vi "LiftSystem.vi"(11 "Lift System Actions":T1) -> ()   [LabVIEW 2019]
uses:
  Controls/Lift System Actions.ctl
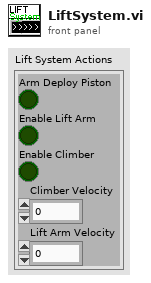
[diagram p1: front panel]
types:
  T1 = typedef "Lift System Actions.ctl" = cluster{"Arm Deploy Piston":bool, "Enable Lift Arm":bool, "Enable Climber":bool, "Climber Velocity":dbl, "Lift Arm Velocity":dbl}
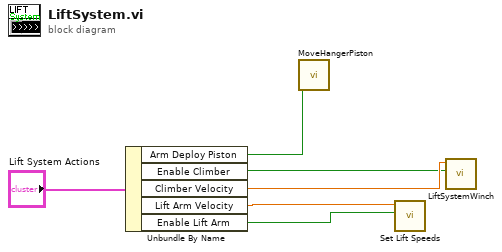
[diagram p0: block diagram]
diagram:
  n1 = Unbundle By Name("Lift System Actions") -> ("Arm Deploy Piston"=w1:bool, "Enable Climber"=w4:bool, "Climber Velocity"=w5:dbl, "Lift Arm Velocity"=w3:dbl, "Enable Lift Arm"=w2:bool)
  n2 = call "MoveHangerPiston.vi"("Arm Deploy Piston"=w1) -> ()  [unwired: 11 in]
  n3 = call "Set Lift Speeds.vi"("Enable Lift Arm"=w2, "Lift Speed"=w3) -> ()  [unwired: 10 in]
  n4 = call "LiftSystemWinch.vi"("Enable"=w4, "climber velocity"=w5) -> ()  [unwired: 10 in]
